vi "FF_Platform.vi"(8 "error in (no error)":errorcluster, 9 "WristVelocity":dbl[](array[numeric]), 10 "WristPosition":dbl[](array[numeric]), 11 "Force Field Controller in":refnum<class "ForceField.lvclass">) -> (0 "error out":errorcluster, 1 "ClosestPt":dbl[](array[numeric]), 2 "Force":dbl[](array[numeric]), 3 "Force Field Controller out":refnum<class "ForceField.lvclass">, 4 "ForceComp":dbl[](array[numeric]))   [LabVIEW 2015, in "ForceField.lvclass"]
uses:
  ForceField.lvclass
  ForceField.lvclass/ForceField.ctl
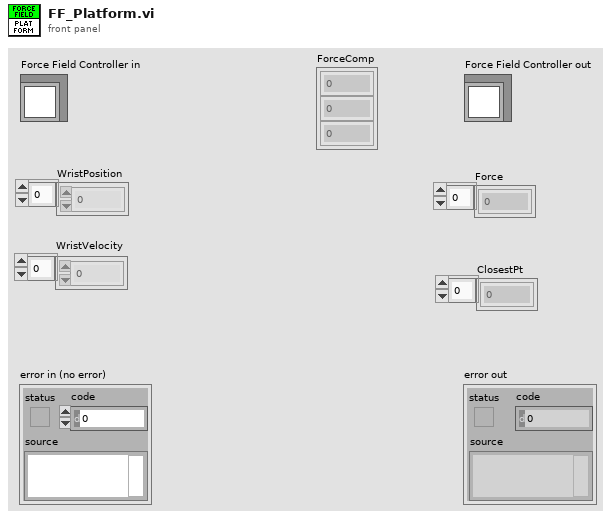
[diagram p1: front panel]
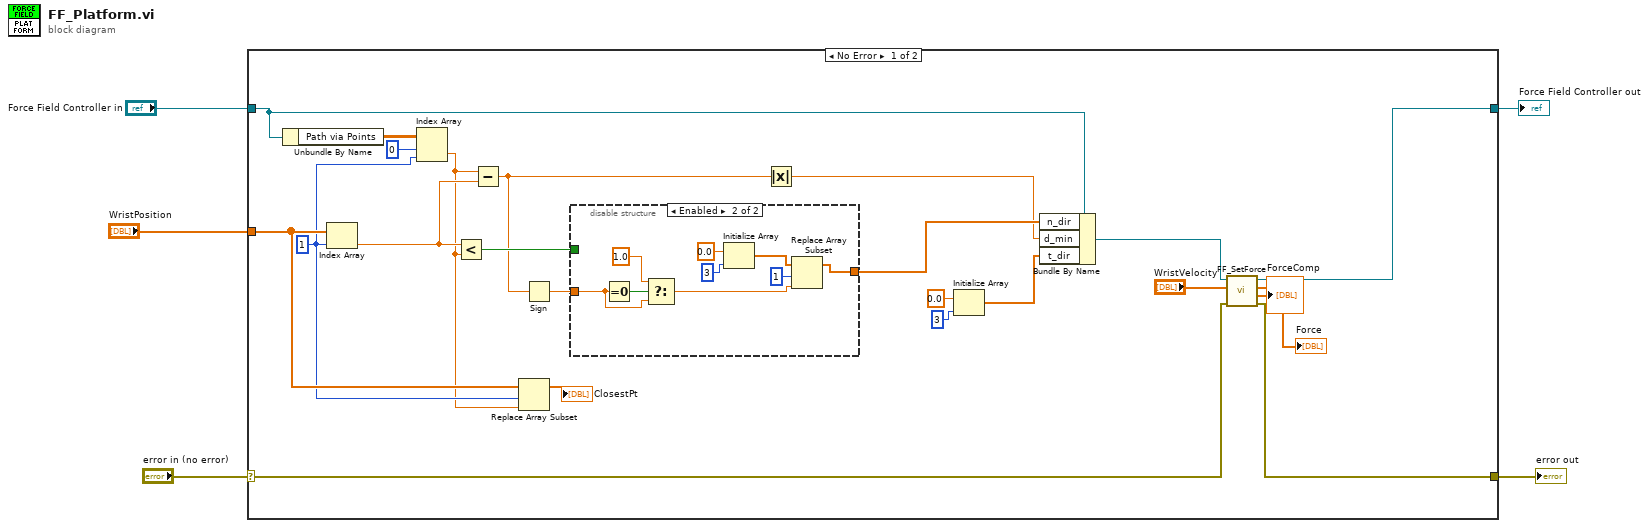
[diagram p0: block diagram]
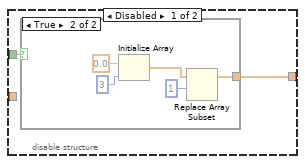
[diagram p2: hidden frame]
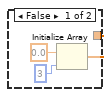
[diagram p3: hidden frame]
diagram:
  n1 = case shown="No Error" "error in (no error)" {
    selector: "error in (no error)" -> [w15 w49]
    tunnel: [w14 w49] -> w4
    tunnel: [w17 w48] -> w2
    tunnel: "Force Field Controller in" -> [w26 w48]
    tunnel: "WristPosition" -> [w10 _]
    frame No Error {
      w9 = 1 ("disabled index (col)")
      n2 = Unbundle By Name(w26) -> ("Path via Points"=w28:dbl[][])
      n3 = Index Array(array=w10, index=w9) -> (element=w23:dbl)
      n4 = Index Array(array=w28, index (row)=0, index (col)=w9) -> (element=w8:dbl)
      n5 = Less?(x=w23, y=w8) -> (x < y?=w25:bool)
      n6 = Subtract(x=w8, y=w23) -> (x-y=w12:dbl)
      n7 = Replace Array Subset(array=w10, new element=w8, index=w9) -> (→"ClosestPt":dbl[])
      n8 = Sign(1:w12) -> (0:w11:dbl)
      n9 = disable-structure shown="Enabled" {
        disable-tunnel: w25 -> [w30 _]
        disable-tunnel: [w29 w43] -> w24
        disable-tunnel: w11 -> [_ w40]
        frame Disabled {
          n10 = case shown="True" w30 {
            tunnel: [w32 w34] -> w29
            frame False {
              n11 = Initialize Array(0.0 ("element"), 3 ("dimension size")) -> (w32:dbl[])
            }
            frame True {
              n12 = Initialize Array(0.0 ("element"), 3 ("dimension size")) -> (w36:dbl[])
              n13 = Replace Array Subset(array=w36, index=1) -> (w34:dbl[])  [unwired: 1 in]
            }
          }
        }
        frame Enabled {
          n14 = Equal To 0?(x=w40) -> (x = 0?=w42:bool)
          n15 = Select(t=1.0, s=w42, f=w40) -> (s? t:f=w41:dbl)
          n16 = Initialize Array(0.0 ("element"), 3 ("dimension size")) -> (w45:dbl[])
          n17 = Replace Array Subset(array=w45, new element=w41, index=1) -> (w43:dbl[])
        }
      }
      n18 = Absolute Value(x=w12) -> (abs(x)=w22:dbl)
      n19 = Initialize Array(0.0 ("element"), 3 ("dimension size")) -> (w20:dbl[])
      n20 = Bundle By Name(cluster=w26, "n_dir"=w24, "d_min"=w22, "t_dir"=w20) -> (w18:refnum<class "ForceField.lvclass">)
      n21 = call "FF_SetForce.vi"("error in (no error)"=w15, "AnkleVelocity"="WristVelocity", "Force Field Controller in"=w18) -> ("error out"=w14:errorcluster, "ForceNTD"=→"ForceComp":dbl[], "ForceXYZ"=→"Force":dbl[], "Force Field Controller out"=w17:refnum<class "ForceField.lvclass">)  [unwired: 5 in]
    }
    frame Error {
    }
  }
  "error out" <- w4
  "Force Field Controller out" <- w2
